vi "saveFreqSweep.vi"(9 "f-res, Hz":dbl, 10 "Frequency Scan":cluster{i32[], "Best Gaussian Fit":dbl[]}[](array[cluster]), 11 "file path (dialog if empty)":path) -> ()   [LabVIEW 2011]
uses:
  <vilib>/Utility/file.llb/Write To Spreadsheet File (string).vi
  <vilib>/Utility/file.llb/Write To Spreadsheet File (DBL).vi
panel:
  # "filename MUST include number, e.g. filename_1.txt"
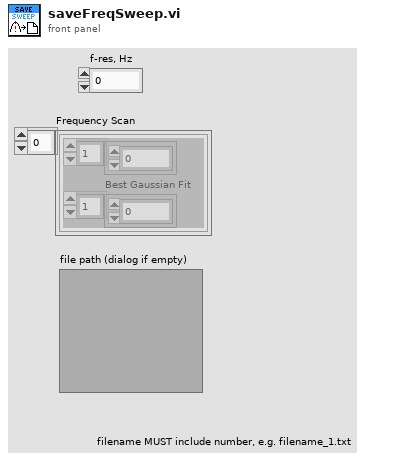
[diagram p1: front panel]
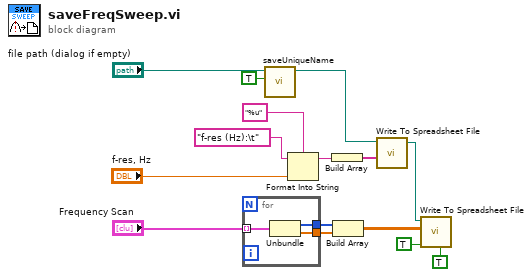
[diagram p0: block diagram]
diagram:
  n1 = for {
    tunnel: "Frequency Scan" -> [w18] mode=indexing
    tunnel: [w17] -> w14
    tunnel: [w16] -> w15
    n2 = Unbundle(w18) -> (w17:i32[], "Best Gaussian Fit"=w16:dbl[])
  }
  n3 = call "saveUniqueName.vi"("Check existence before modifying path"=TRUE, "path"="file path (dialog if empty)") -> ("unique path"=w3:path)  [unwired: 8 in, 1 out]
  n4 = Format Into String(format string="%u" ("%u"), initial string="f-res (Hz):\t" ("%u"), "f-res, Hz") -> (resulting string=w5:string)  [unwired: 1 in, 1 out]
  n5 = Build Array(w5) -> (w4:string[])
  n6 = Build Array(w14, w15) -> (w8:dbl[][])
  n7 = call-poly <vilib>:"Write To Spreadsheet File.vi"("1D data"=w4, "file path (dialog if empty)"=w3) -> ("new file path (Not A Path if cancelled)"=w2:path)  [unwired: 6 in]
  n8 = call-poly <vilib>:"Write To Spreadsheet File.vi"("transpose? (no:F)"=TRUE, "append to file? (new file:F)"=TRUE, "2D data"=w8, "file path (dialog if empty)"=w2) -> ()  [unwired: 4 in, 1 out]
